vi "subVI_Init&GetParams.vi"(2 "Mono2 Pos":refnum<vi>, 3 "Mono2 Velocity":refnum<vi>) -> (1 "Mono2 On":bool caption="Motor On?")   [LabVIEW 2019]
uses:
  Globals/InstrumentReferences.vi
panel:
  in  "ESP300 Error":errorcluster
  in  "Mono2 Motor Pos":dbl caption="Motor Pos"
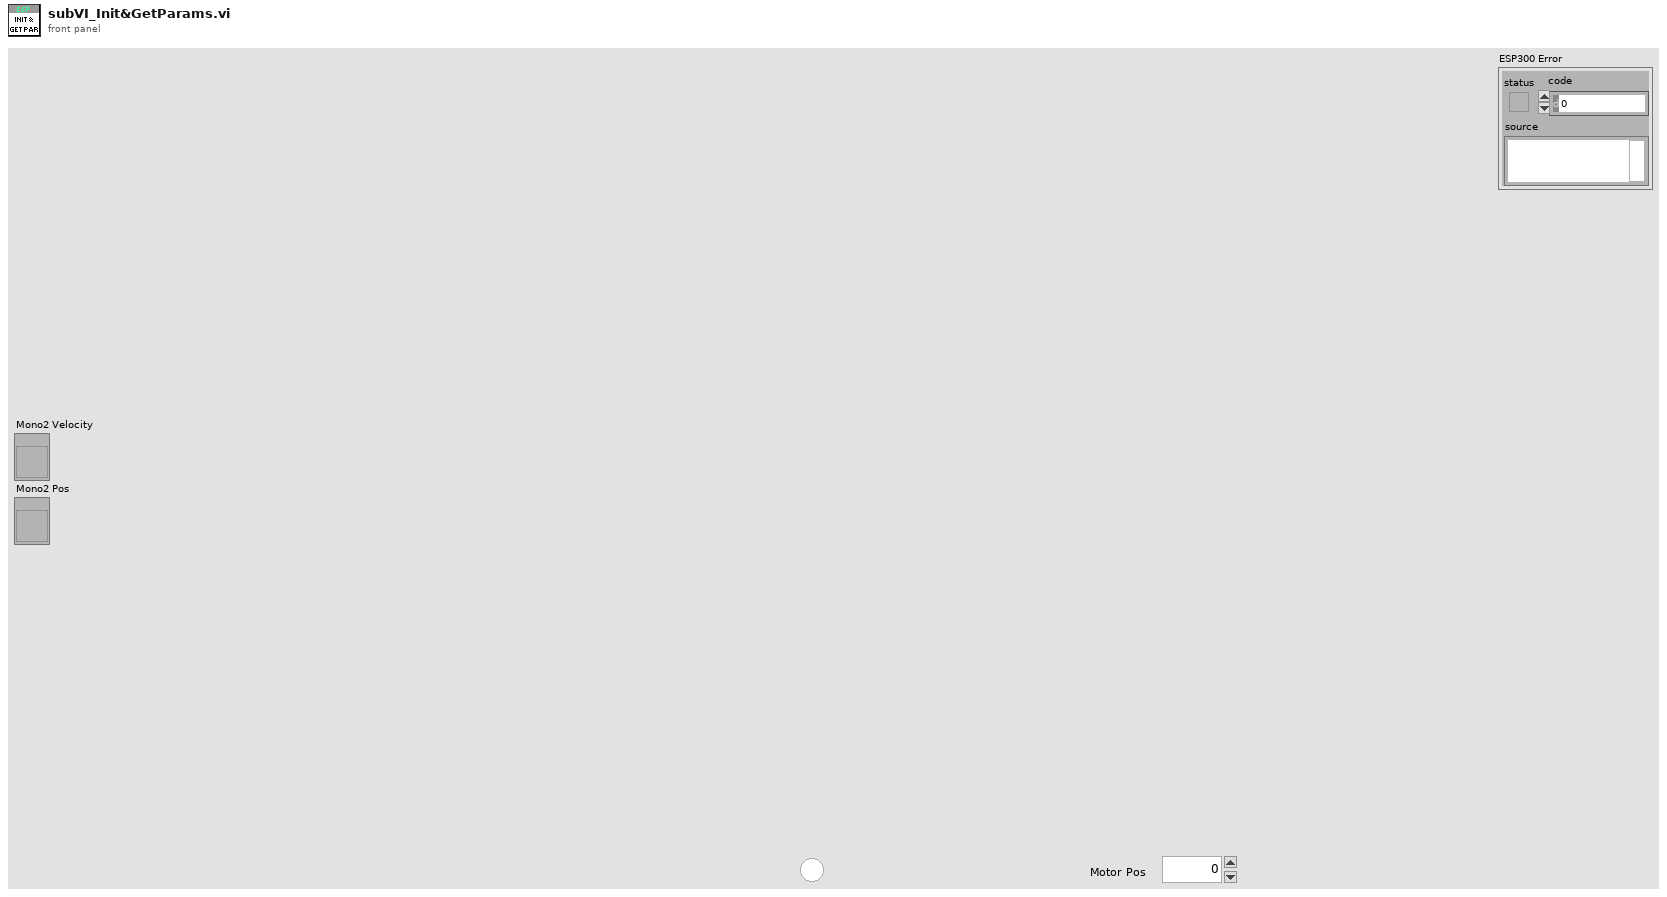
[diagram p1: front panel]
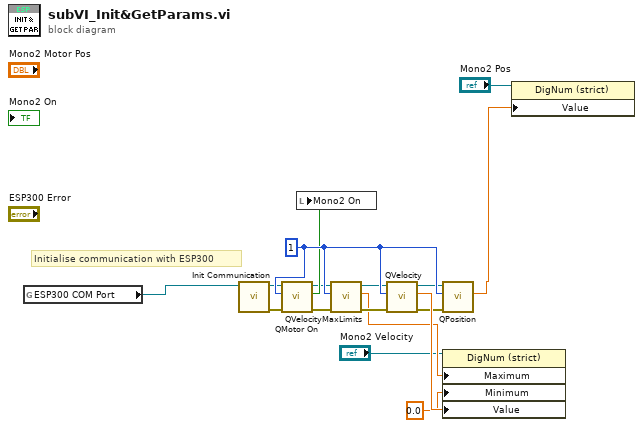
[diagram p0: block diagram]
diagram:
  w16 = 1 ("Axis")
  # "Initialise communication with ESP300"
  n1 = global read "InstrumentReferences.vi" "ESP300 COM Port"() -> (w1:refnum<visa-resource-name>)
  n2 = call "Init Communication.vi"("VISA resource name in"=w1) -> ("error out"=w6:errorcluster, "VISA resource name out"=w5:refnum<visa-resource-name>)  [unwired: 9 in]
  n3 = call "QMotor On.vi"("error in (no error)"=w6, "Axis"=w16, "VISA resource name in"=w5) -> ("error out"=w8:errorcluster, "Motor On?"=w9:bool, "VISA resource name out"=w7:refnum<visa-resource-name>)  [unwired: 6 in]
  n4 = local write "Mono2 On"(w9) -> ()
  n5 = call "QVelocityMaxLimits.vi"("error in (no error)"=w8, "Axis"=w16, "VISA resource name in"=w7) -> ("error out"=w13:errorcluster, "Velocity"=w10:dbl, "VISA resource name out"=w12:refnum<visa-resource-name>)  [unwired: 6 in]
  n6 = call "QVelocity.vi"("error in (no error)"=w13, "Axis"=w16, "VISA resource name in"=w12) -> ("error out"=w15:errorcluster, "Velocity"=w17:dbl, "VISA resource name out"=w14:refnum<visa-resource-name>)  [unwired: 6 in]
  n7 = call "QPosition.vi"("error in (no error)"=w15, "Axis"=w16, "VISA resource name in"=w14) -> ("Position"=w2:dbl)  [unwired: 6 in, 2 out]
  n8 = property on="Property Node" class="DigNum (strict)"(reference="Mono2 Velocity", "Maximum"=w10, "Minimum"=0.0 ("Data Entry Limits:Minimum"), "Value"=w17) -> ()  [unwired: 1 in, 2 out]
  n9 = property on="Property Node" class="DigNum (strict)"(reference="Mono2 Pos", "Value"=w2) -> ()  [unwired: 1 in, 2 out]
